vi "Support_AddResult.vi"(2 "Results in":T1[](array[typedef]) {"MeasurementValue" format="%.2f"}, 3 "Pass":bool, 4 "Comment":string, 5 "MeasurementValue":dbl format="%.2f", 7 "Pass comment":string, 9 "Fail comment":string) -> (16 "Results out":T1[](array[typedef]) {"MeasurementValue" format="%.2f"})   [LabVIEW 2017]
doc: "Adds to result."
uses:
  Support_ResultType.ctl
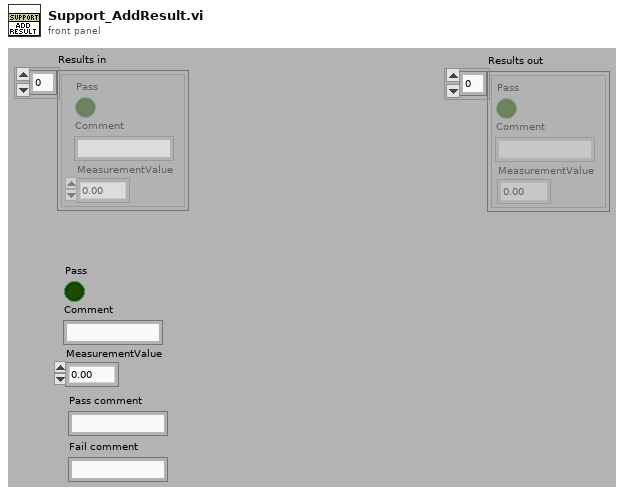
[diagram p1: front panel]
types:
  T1 = typedef "Support_ResultType.ctl" = cluster{"Pass":bool, "Comment":string, "MeasurementValue":dbl}
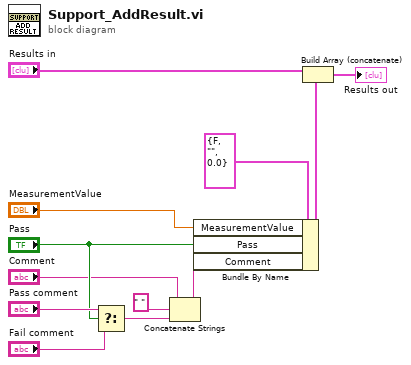
[diagram p0: block diagram]
diagram:
  n1 = Select(t="Pass comment", s="Pass", f="Fail comment") -> (s? t:f=w4:string)
  n2 = Concatenate Strings("Comment", " ", w4) -> (w2:string)
  n3 = Bundle By Name(cluster=T1 {"Pass"=FALSE, "Comment"="", "MeasurementValue"=0.0} ("ResultType"), "MeasurementValue"="MeasurementValue", "Pass"="Pass", "Comment"=w2) -> (w10:T1)
  n4 = Build Array (concatenate)("Results in", w10) -> (→"Results out":T1[])
